vi "Wait For DO Signal Bank.vi"(8 "error in (no error)":errorcluster, 10 "timeout (ms)":i32=5000, 11 "Desired Fresh State":bool) -> (0 "error out":errorcluster={"status"=TRUE, "code"=555, "source"="Timed out waiting for Signal Bank."})   [LabVIEW 2020]
uses:
  PXI Globals.vi
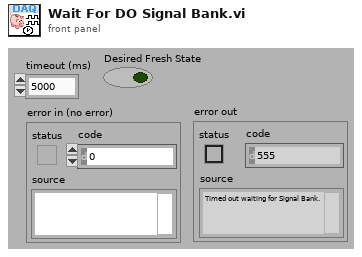
[diagram p1: front panel]
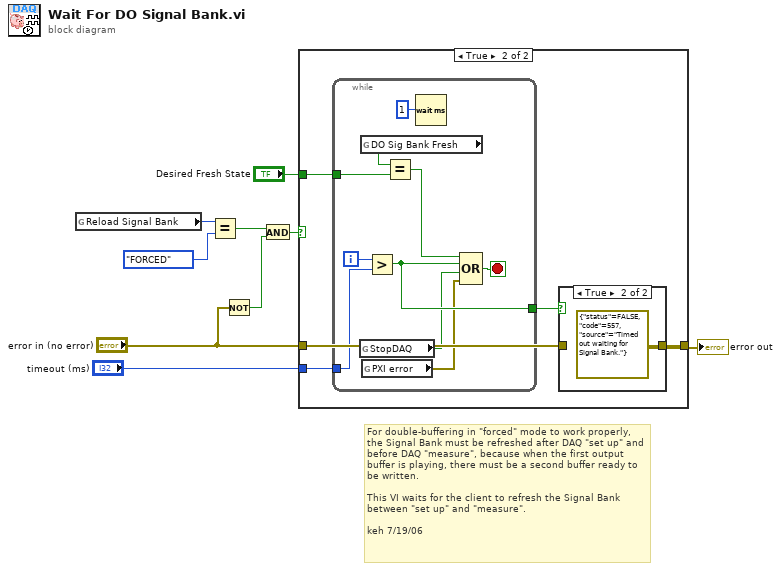
[diagram p0: block diagram]
diagram:
  # "For double-buffering in \"forced\" mode to work properly, the Signal Bank must be refreshed after DAQ \"set up\" and before DAQ \"measure\", because when the first output buffer is playing, there must be a second buffer ready to be written. \n\nThis VI waits for the client to refresh the Signal Bank between \"set up\" and \"measure\".\n\nkeh 7/19/06"
  n1 = global read "PXI Globals.vi" "Reload Signal Bank"() -> (w9:enum32{"OFF", "ENABLED", "FORCED"})
  n2 = Equal?(x=w9, y=enum16{"OFF", "ENABLED", "FORCED"}."FORCED") -> (x = y?=w3:bool)
  n3 = Not(x="error in (no error)") -> (.not. x?=w6:bool)
  n4 = And(x=w3, y=w6) -> (x .and. y?=w5:bool)
  n5 = case shown="True" w5 {
    tunnel: "error in (no error)" -> [w10 w14]
    tunnel: [w10 w13] -> w7
    tunnel: "timeout (ms)" -> [_ w12]
    tunnel: "Desired Fresh State" -> [_ w11]
    frame False {
    }
    frame True {
      n6 = while {
        tunnel: w12 -> [w23]
        tunnel: [w24] -> w15
        tunnel: w11 -> [w20]
        i -> [w25]
        stop <- w26 stop-if-true
        n7 = global read "PXI Globals.vi" "StopDAQ"() -> (w22:bool)
        n8 = global read "PXI Globals.vi" "DO Sig Bank Fresh"() -> (w21:bool)
        n9 = global read "PXI Globals.vi" "PXI error"() -> (w18:errorcluster)
        n10 = Greater?(x=w25, y=w23) -> (0:w24:bool)
        n11 = Equal?(x=w21, y=w20) -> (x = y?=w19:bool)
        n12 = Wait (ms)(milliseconds to wait=1) -> ()  [unwired: 1 out]
        n13 = Compound Arithmetic op=OR(w19, w24, w22, w18) -> (w26:bool)
      }
      n14 = case shown="True" w15 {
        tunnel: w14 -> [w16 _]
        tunnel: [w16 errorcluster {"status"=FALSE, "code"=557, "source"="Timed out waiting for Signal Bank."} ("error out 2")] -> w13
        frame False {
        }
        frame True {
        }
      }
    }
  }
  "error out" <- w7
